vi "BL_GetMessage.vi"(8 "error in (no error)":errorcluster, 10 "Channel":u8, 11 "Potentiostat Galvanostat in":refnum<class "Potentiostat Galvanostat.lvclass">) -> (0 "error out":errorcluster, 1 "Message":string, 2 "Channel":u8, 3 "Potentiostat Galvanostat out":refnum<class "Potentiostat Galvanostat.lvclass">)   [LabVIEW 2018, in "Potentiostat Galvanostat.lvclass"]
doc: "This function copies into the buffer the messages generated by the\nfirmware of selected channel. Be aware that messages are retrieved\none-by-one, this implies this function must be called several times in\norder to get all messages available in the message queue."
uses:
  Potentiostat Galvanostat.lvclass
  Potentiostat Galvanostat.lvclass/Potentiostat Galvanostat.ctl
  BL_GetErrorMsg.vi
  <vilib>/Utility/error.llb/Error Cluster From Error Code.vi
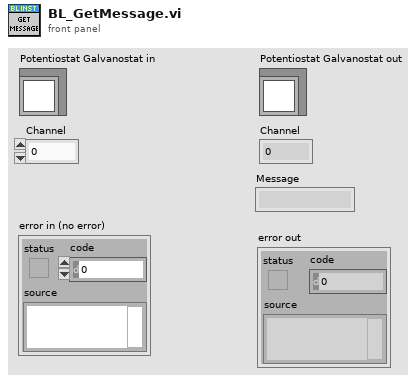
[diagram p1: front panel]
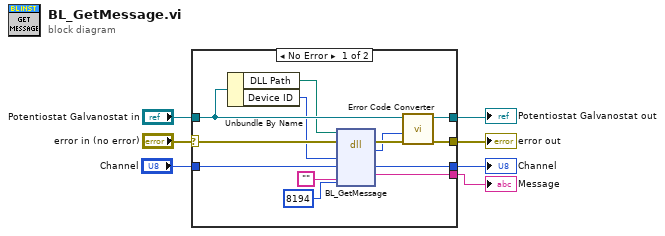
[diagram p0: block diagram]
diagram:
  n1 = case shown="No Error" "error in (no error)" {
    selector: "error in (no error)" -> [w14 w22]
    tunnel: [w20 w22] -> w6
    tunnel: [w19 w21] -> w4
    tunnel: "Potentiostat Galvanostat in" -> [w18 w21]
    tunnel: "Channel" -> [w13 _]
    tunnel: [w9 _] -> w1
    tunnel: [w8 _] -> w2
    frame No Error {
      n2 = Unbundle By Name(w18) -> ("DLL Path"=w12:path, "Device ID"=w11:i32)
      n3 = dll-call lib="C:/Program Files (x86)/National Instruments/LabVIEW 2018/user.lib/EClib/EClib.*" fn="BL_GetMessage"(path in=w12, error in=w14, "Device ID"=w11, "Channel"=w13, "Message"="", "Size"=u32 8194) -> (error out=w15:errorcluster, "Error Code"=w10:i32, "Channel"=w8:u8, "Message"=w9:string)  [unwired: 3 in, 1 out]
      n4 = call "Error Code Converter.vi"("error in (no error)"=w15, "Error Code"=w10, "Potentiostat Galvanostat in"=w18) -> ("error out"=w20:errorcluster, "Potentiostat Galvanostat out"=w19:refnum<class "Potentiostat Galvanostat.lvclass">)  [unwired: 7 in]
    }
    frame Error {
    }
  }
  "error out" <- w6
  "Potentiostat Galvanostat out" <- w4
  "Channel" <- w2
  "Message" <- w1
